vi "禹山浊度校准.vi"() -> ()   [LabVIEW 2016, in "斯坦道多参数.lvlib"]
uses:
  <vilib>/Utility/miscctls.llb/LVPointTypeDef.ctl
  <vilib>/Analysis/NI_AALBase.lvlib
  <vilib>/Analysis/NI_AALPro.lvlib
  <vilib>/Utility/config.llb/NI_LVConfig.lvlib
panel:
  out "滤波设定":dbl
  out "通讯状态":string
  out "第二点校准值":dbl
  out "第一点校准值":dbl
  out "最小值":sgl format="%.2g"
  out "最大值":sgl format="%.2g"
  in  "校准停止":bool
  in  "校准模式":u16(ring) items=["两点校准", "单点校准"]
  in  "标液2":dbl
  in  "标液1":dbl
  out "波形图表":sgl(graph) caption="历史曲线"
  out "温度测量值":dbl caption="温度" format="%#.2f"
  out "变异系数":dbl format="%.6g"
  out "standard deviation":dbl caption="标准差" format="%0.2f"
  out "mean":dbl caption="均值" format="%0.2f"
  out "提示":string
  in  "校准启动":bool
  out "测试值":dbl format="%#.2f"
  out "电极斜率":dbl format="%#.6f"
  out "电极零点":dbl format="%#.6f"
  # "浊度电极设定"
  # "℃"
  # "NTU"
  # "请选择校准模式:"
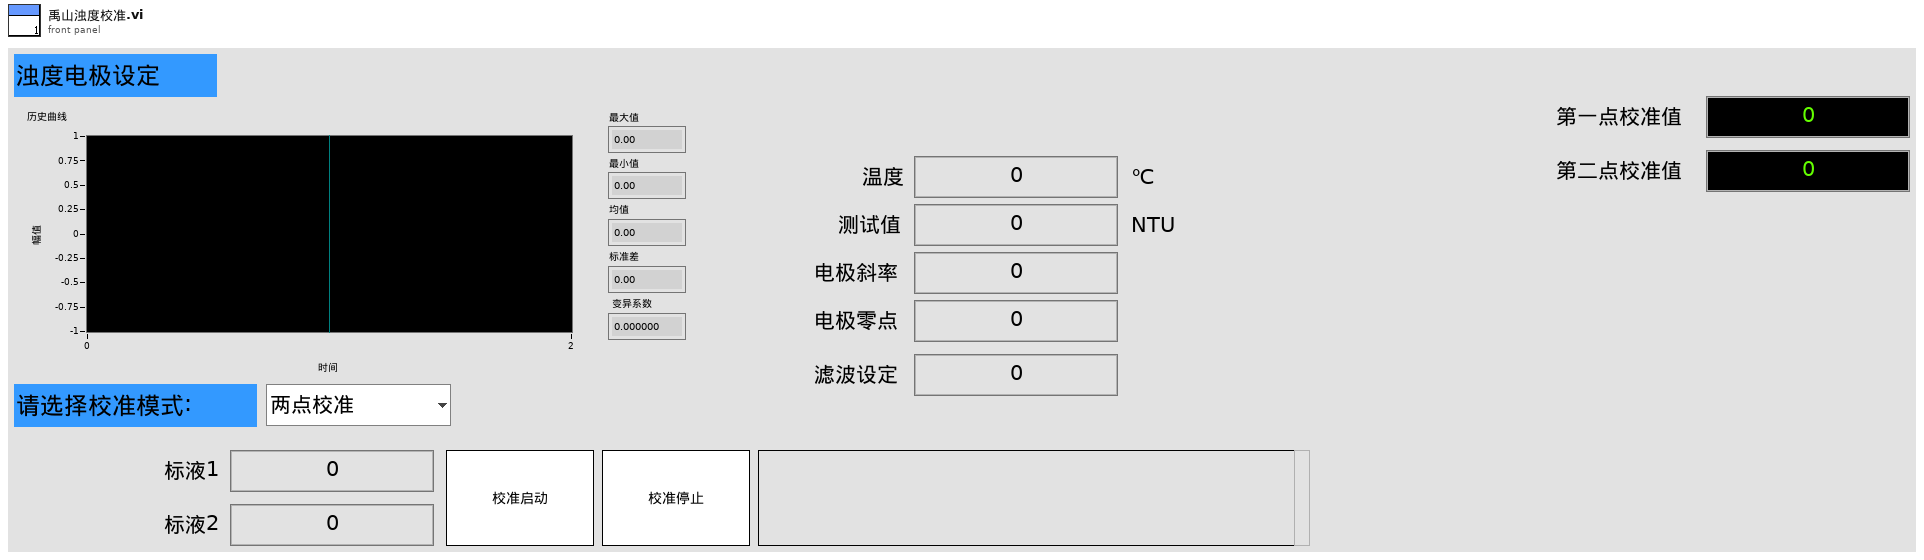
[diagram p1: front panel]
types:
  T1 = typedef "LVPointTypeDef.ctl" = cluster{"Horizontal":i16, "Vertical":i16}
  T2 = cluster{"pH":u32, "DO":u32, "Cond":u32, "Turb":u32, "叶绿素a":u32, "藻密度":u32, "ORP":u32}
  T3 = typedef "NI_LVConfig.lvlib/Config Data RefNum.ctl" = refnum<k1>
  T4 = enum8{"Enabled", "Disabled", "Disabled and Grayed Out"}
  T5 = cluster{"ph":bool, "DO":bool, "Cond":bool, "Turb":bool, "叶绿素a":bool, "藻密度":bool, "ORP":bool}
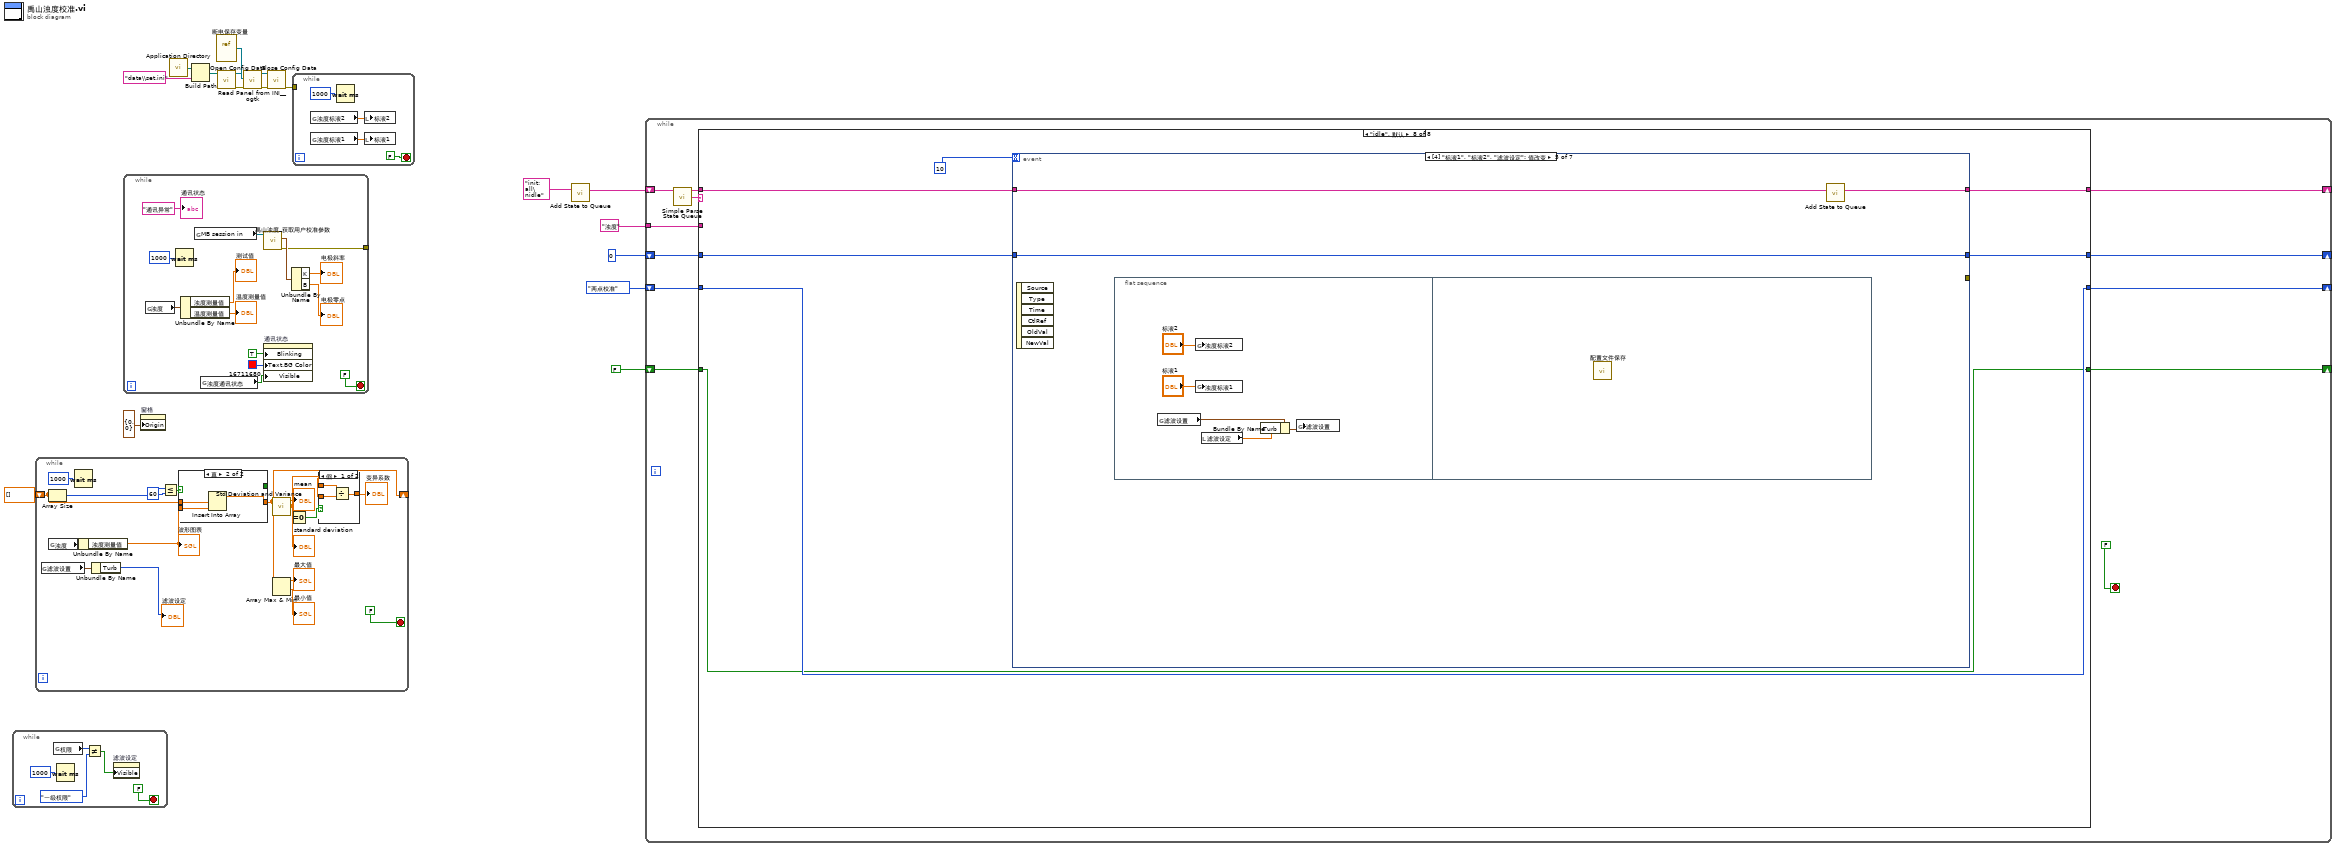
[diagram p0: block diagram]
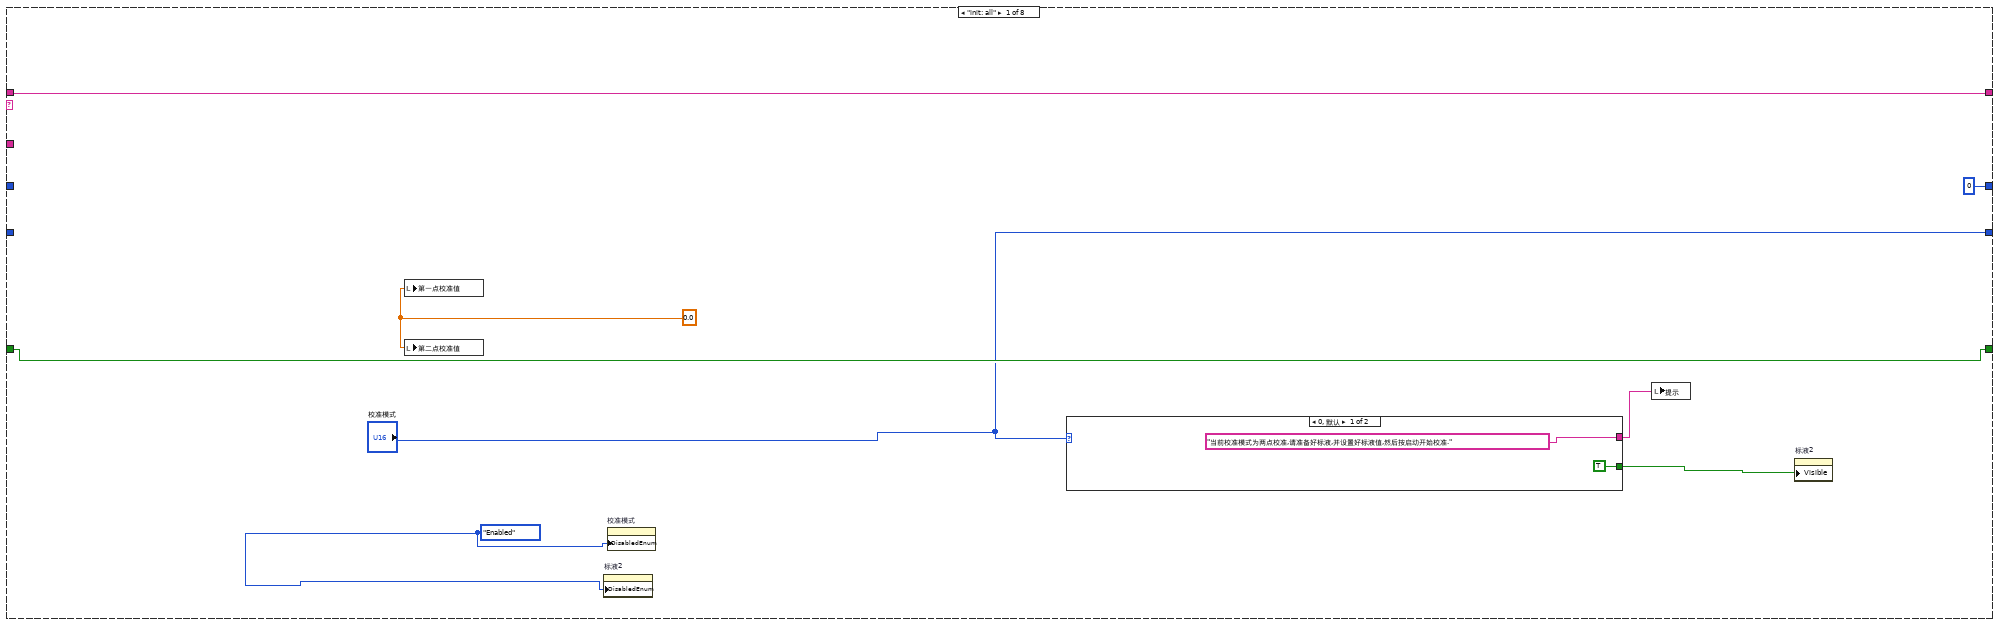
[diagram p2: hidden frame]
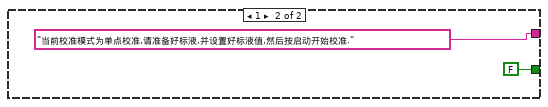
[diagram p3: hidden frame]
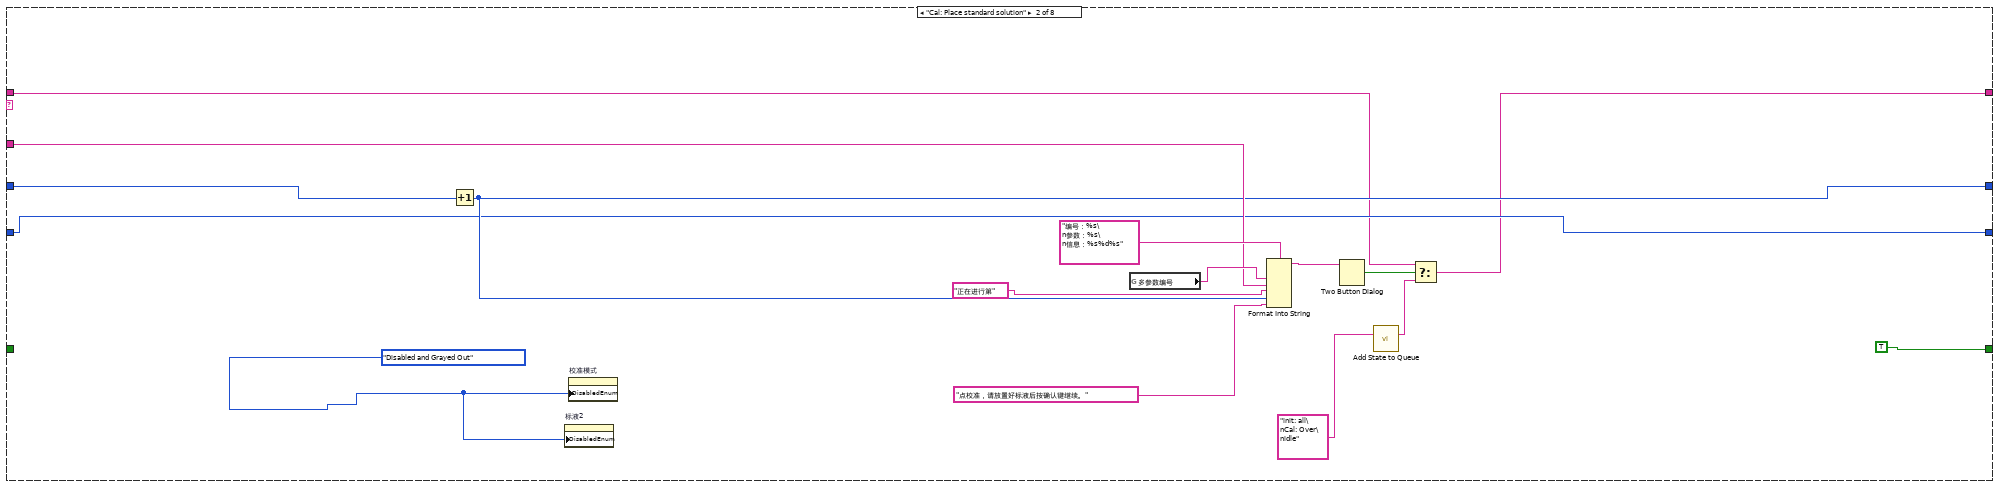
[diagram p4: hidden frame]
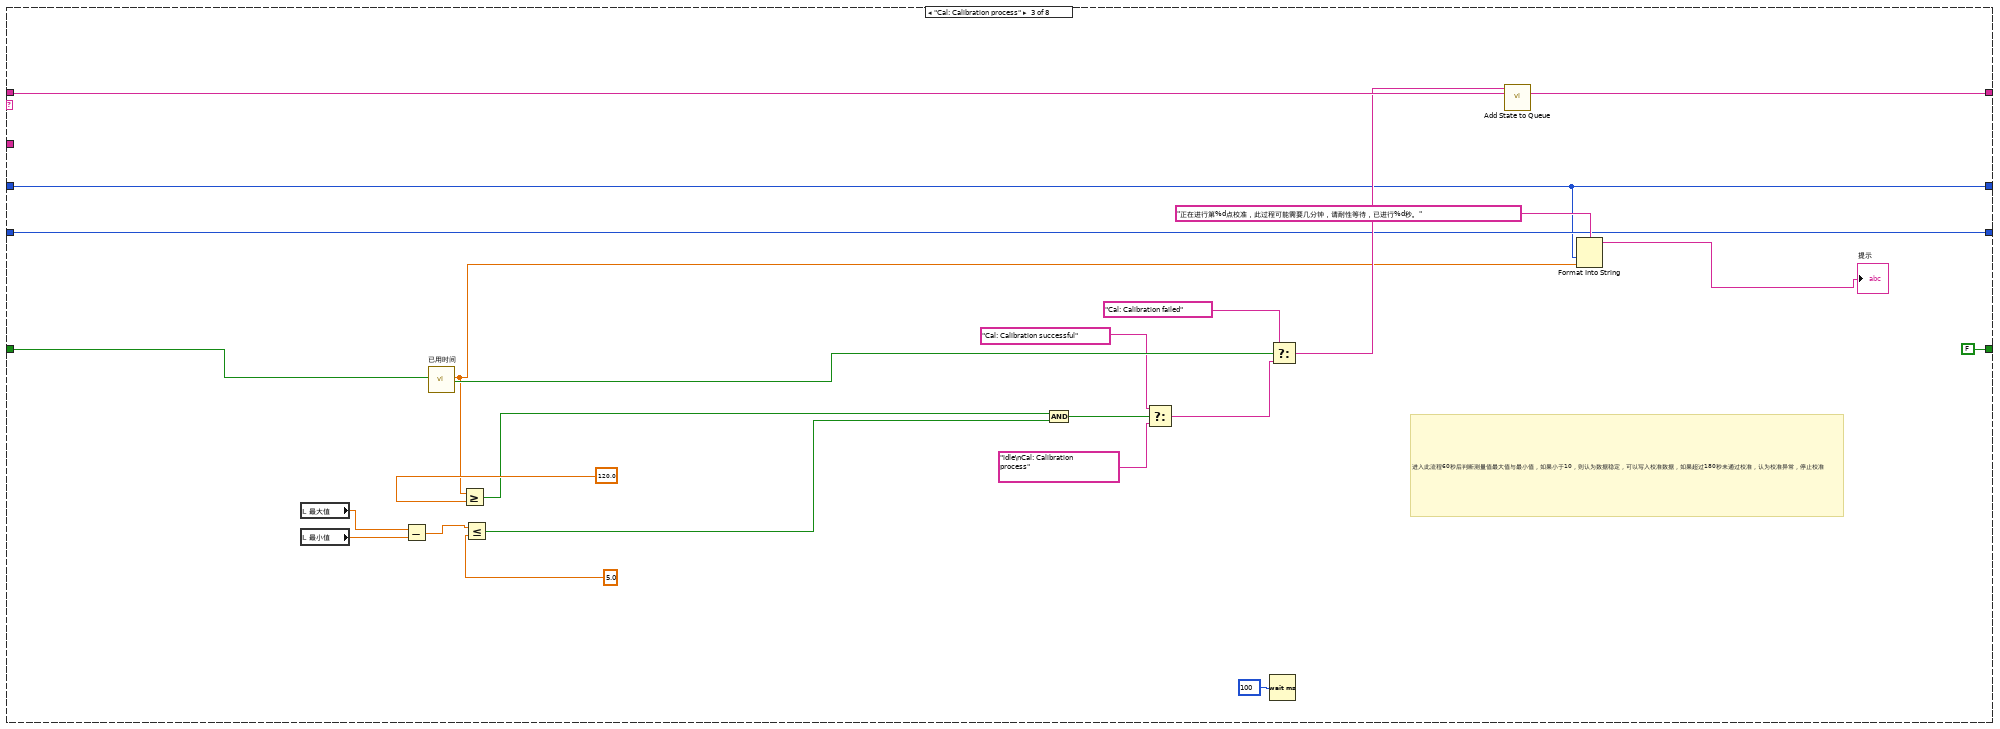
[diagram p5: hidden frame]
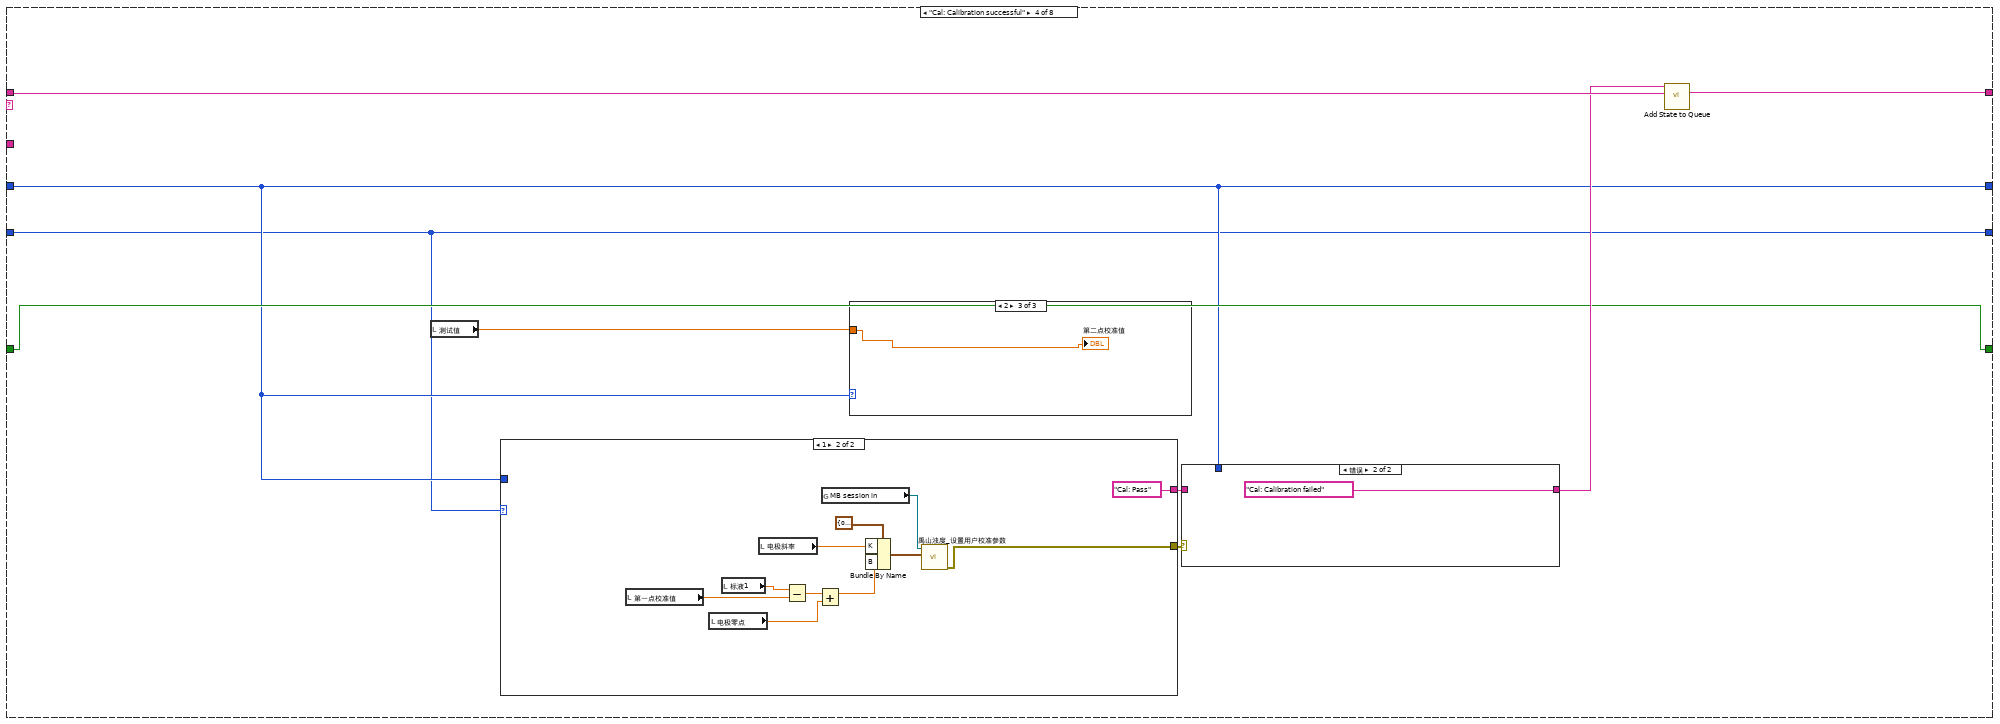
[diagram p6: hidden frame]
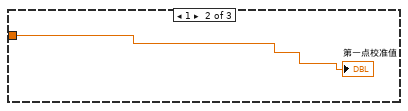
[diagram p8: hidden frame]
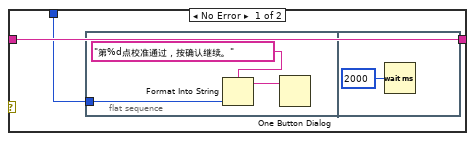
[diagram p9: hidden frame]
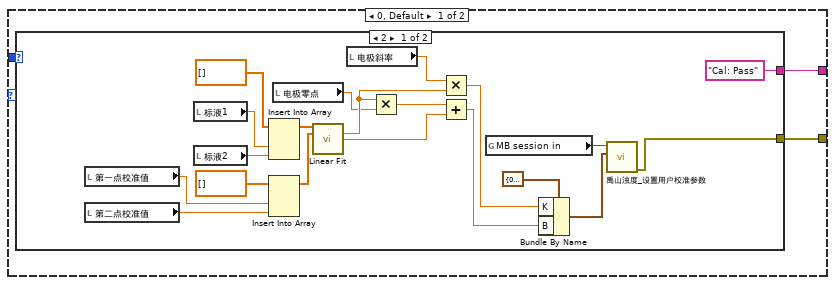
[diagram p10: hidden frame]
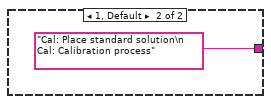
[diagram p11: hidden frame]
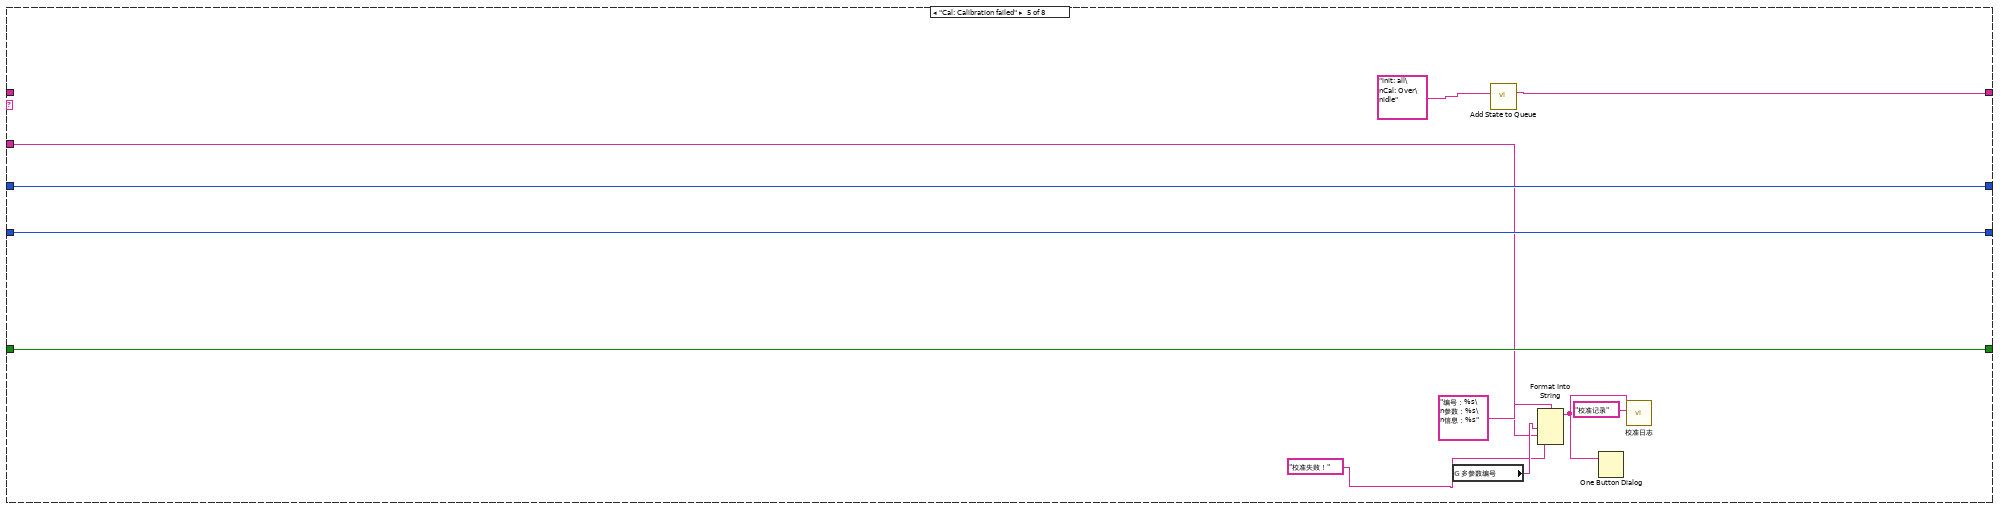
[diagram p12: hidden frame]
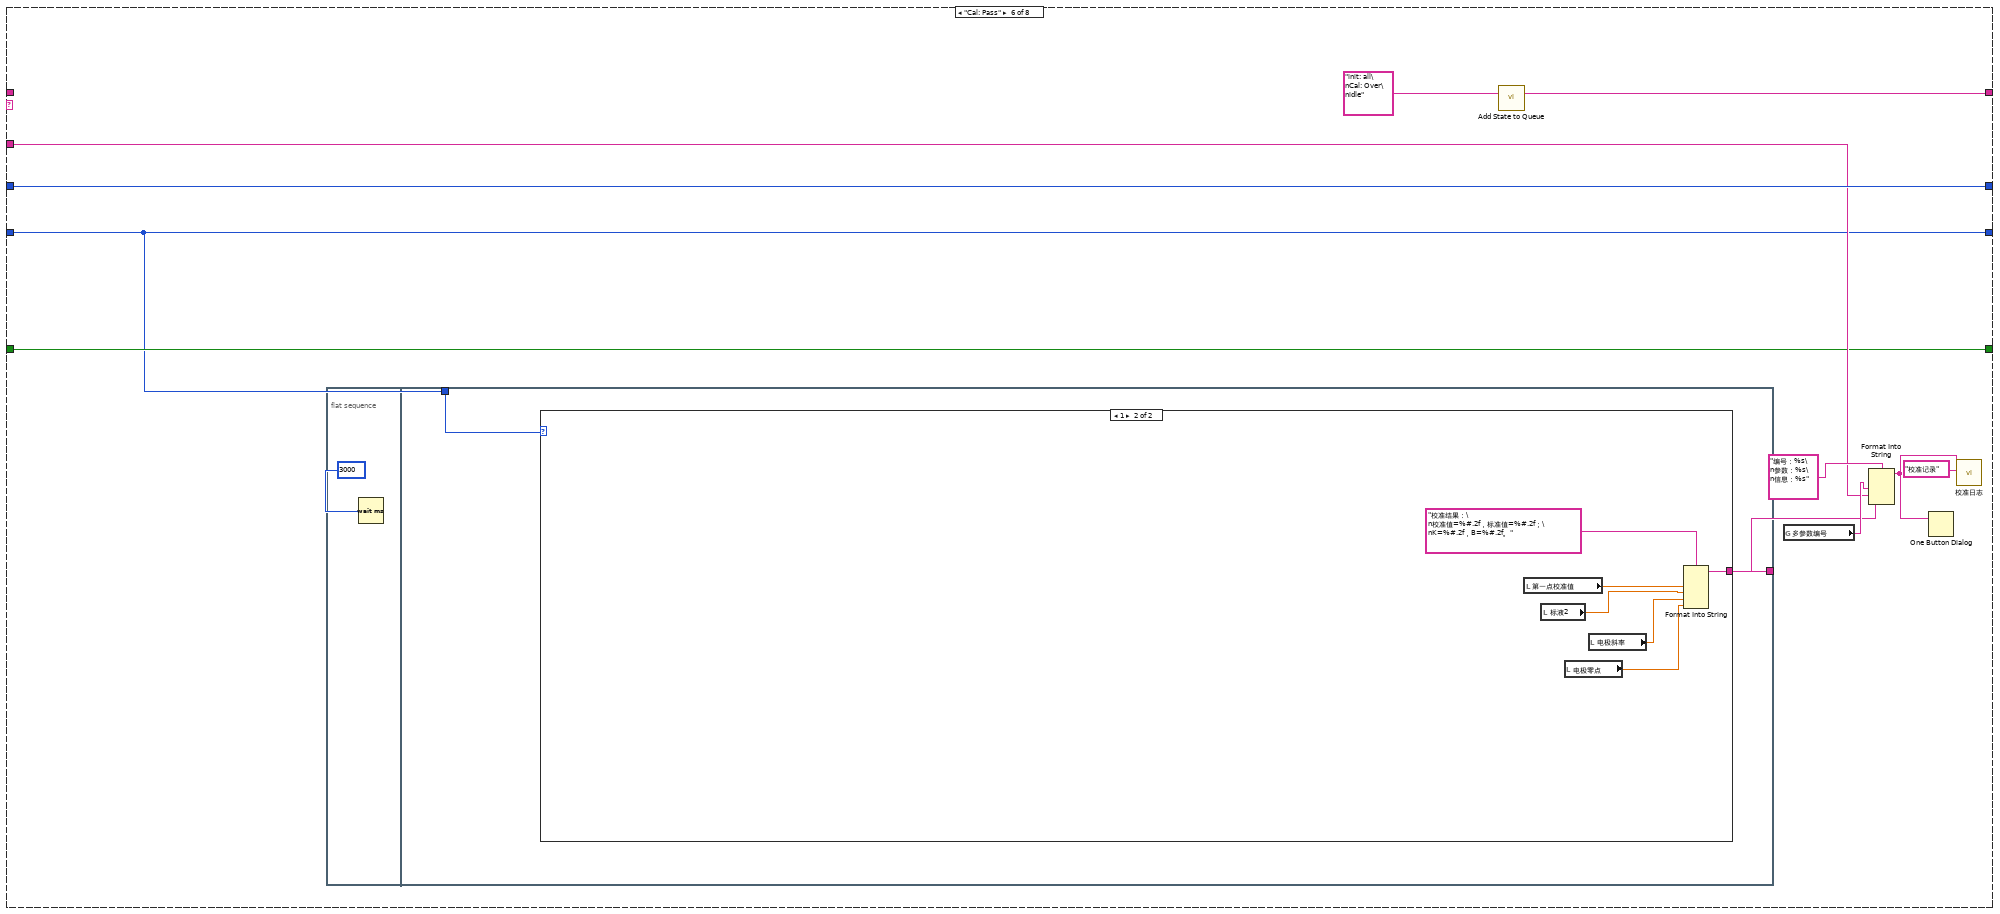
[diagram p13: hidden frame]
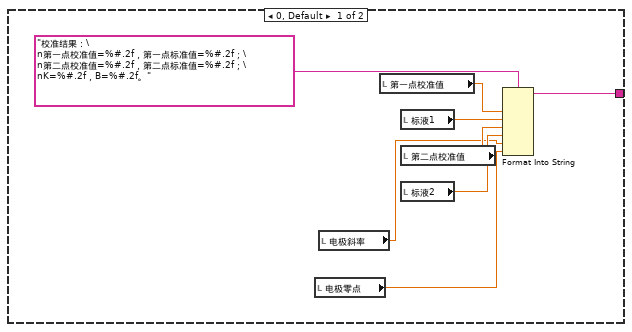
[diagram p14: hidden frame]
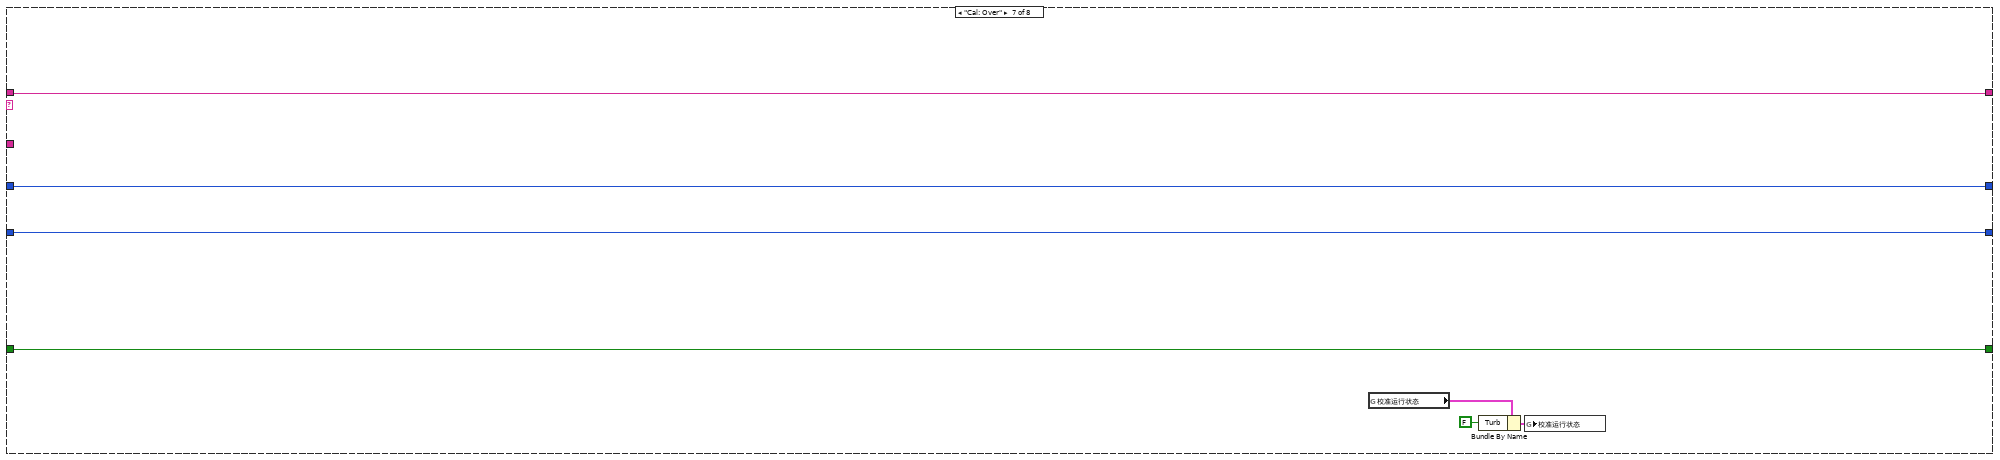
[diagram p15: hidden frame]
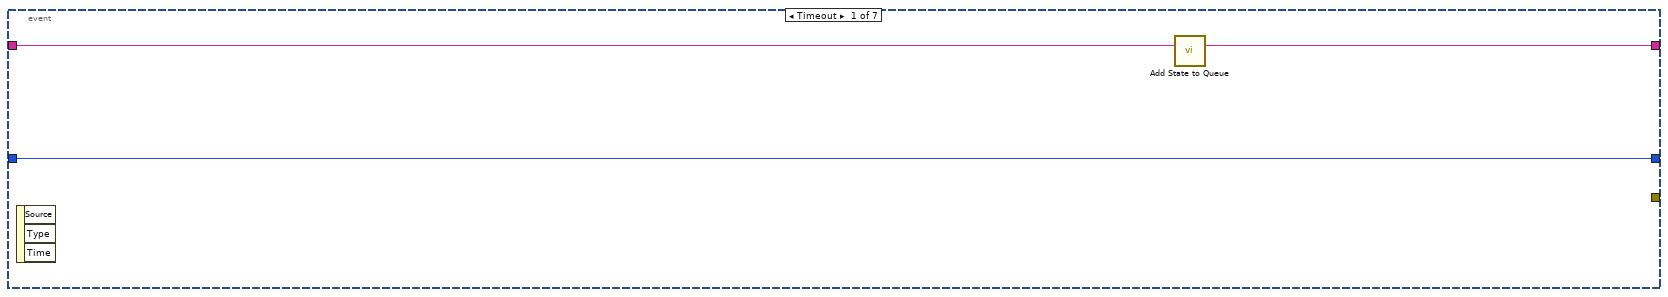
[diagram p16: hidden frame]
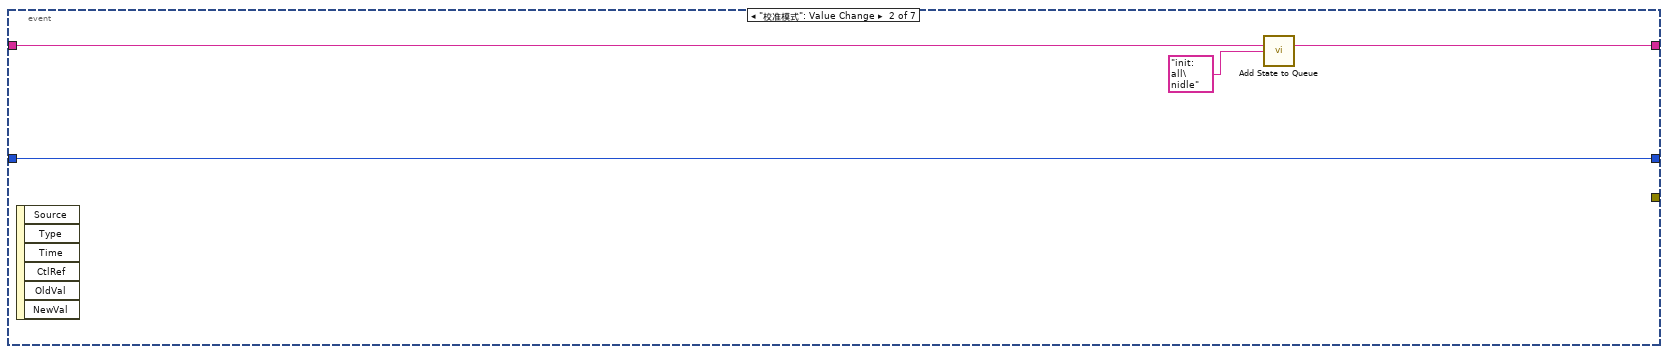
[diagram p17: hidden frame]
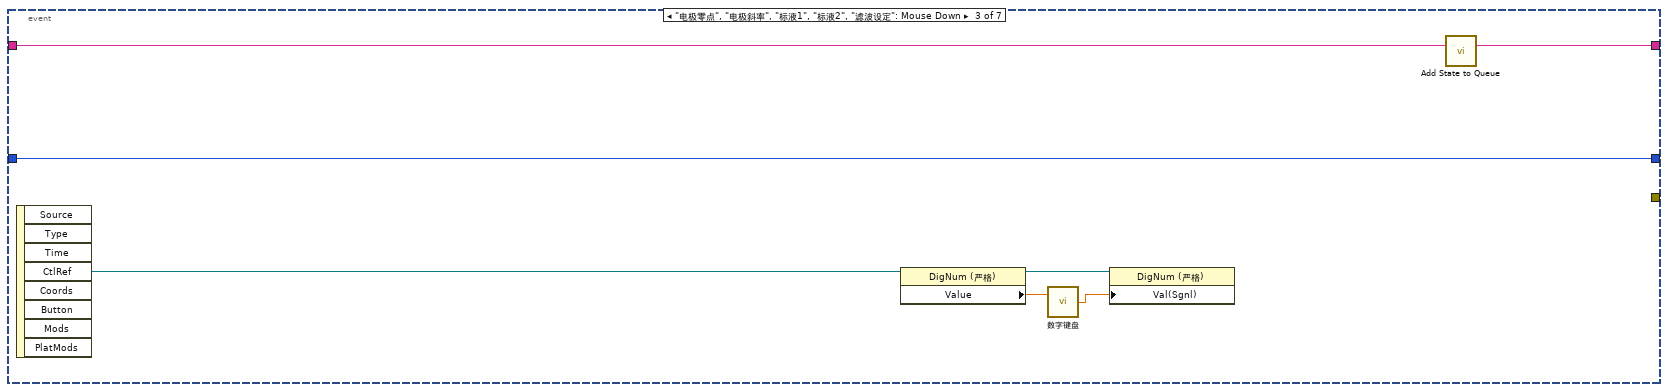
[diagram p18: hidden frame]
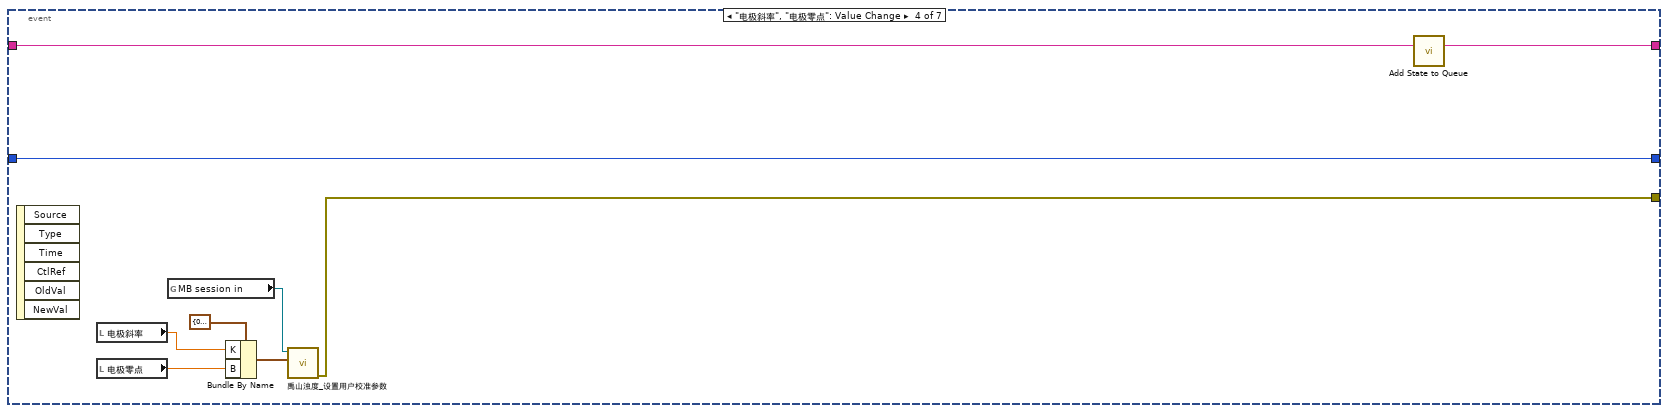
[diagram p19: hidden frame]
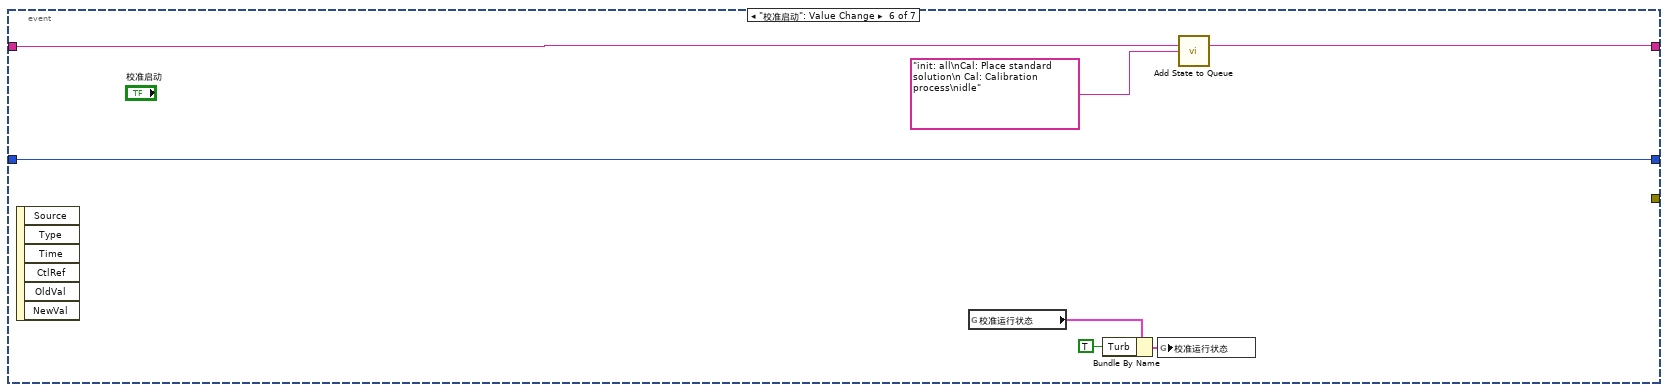
[diagram p20: hidden frame]
diagram:
  n1 = while {
    stop <- FALSE stop-if-true
    n2 = global read "多参数全局变量.vi" "权限"() -> (w21:enum16{"一级权限", "二级权限", "三级权限"})
    n3 = Wait (ms)(milliseconds to wait=u32 1000 ("等待时间（毫秒）")) -> ()  [unwired: 1 out]
    n4 = Not Equal?(x=w21, y=enum16{"一级权限", "二级权限", "三级权限"}."一级权限") -> (x != y?=w18:bool)
    n5 = property on="滤波设定" class="DigNum (严格)"("Visible"=w18) -> ()  [unwired: 2 in, 2 out]
  }
  n6 = while {
    shift-right: [w28] -> _
    shift-left: sgl[] [] -> [w35]
    stop <- FALSE stop-if-true
    n7 = global read "断电保存变量.vi" "滤波设置"() -> (w24:T2)
    n8 = Array Size(array=w35) -> (size(s)=w37:i32)
    n9 = global read "禹山过程全局变量.vi" "浊度"() -> (w29:cluster{"温度测量值":sgl, "浊度测量值":sgl})
    n10 = Wait (ms)(milliseconds to wait=u32 1000 ("等待时间（毫秒）")) -> ()  [unwired: 1 out]
    n11 = Unbundle By Name(w29) -> ("浊度测量值"=w25:sgl)
    "波形图表" <- w25
    n12 = Unbundle By Name(w24) -> ("Turb"=→"滤波设定":u32)
    n13 = Less Or Equal?(x=w37, y=60) -> (x <= y?=w36:bool)
    n14 = case shown="真" w36 {
      tunnel: w35 -> [w48 w51]
      tunnel: w25 -> [w46 w50]
      tunnel: [w44 w49] -> w28
      tunnel: [TRUE _] -> _
      frame False {
        n15 = Replace Array Subset(array=w48, new element=w46) -> (w47:sgl[])  [unwired: 1 in]
        n16 = Rotate 1D Array(1:w47, 2:-1 ("n")) -> (0:w44:sgl[])
      }
      frame True {
        n17 = Insert Into Array(array=w51, new element=w50) -> (w49:sgl[])  [unwired: 1 in]
      }
    }
    n18 = call <vilib>:"Std Deviation and Variance.vi"("X"=w28) -> ("mean"=w30:dbl, "standard deviation"=w31:dbl)  [unwired: 1 in, 1 out]
    "standard deviation" <- w31
    "mean" <- w30
    n19 = Array Max & Min(array=w28) -> (max value=→"最大值":sgl, min value=→"最小值":sgl)  [unwired: 2 out]
    n20 = Equal To 0?(x=w30) -> (x = 0?=w34:bool)
    n21 = case shown="假" w34 {
      tunnel: w31 -> [w42 _]
      tunnel: [w41 _] -> w33
      tunnel: w30 -> [w40 _]
      frame False {
        n22 = Divide(x=w42, y=w40) -> (x/y=w41:dbl)
      }
      frame True {
      }
    }
    "变异系数" <- w33
  }
  n23 = while {
    tunnel: [w60] -> _
    stop <- FALSE stop-if-true
    n24 = global read "禹山过程全局变量.vi" "浊度"() -> (w57:cluster{"温度测量值":sgl, "浊度测量值":sgl})
    n25 = Wait (ms)(milliseconds to wait=u32 1000 ("等待时间（毫秒）")) -> ()  [unwired: 1 out]
    n26 = Unbundle By Name(w57) -> ("浊度测量值"=→"测试值":sgl, "温度测量值"=→"温度测量值":sgl)
    n27 = global read "多参数全局变量.vi" "MB session in"() -> (w56:refnum<class "MB_Master.lvclass">)
    n28 = global read "多参数全局变量.vi" "浊度通讯状态"() -> (w52:bool)
    n29 = call "禹山浊度_获取用户校准参数.vi"("MB session in"=w56) -> ("error out"=w60:errorcluster, "输出值"=w63:cluster{"K":sgl, "B":sgl})  [unwired: 8 in, 1 out]
    n30 = property on="通讯状态" class="Str"("Blinking"=TRUE ("闪烁"), "Text.BG Color"=u32 16711680, "Visible"=w52) -> ()  [unwired: 2 in, 2 out]
    n31 = Unbundle By Name(w63) -> ("K"=→"电极斜率":sgl, "B"=→"电极零点":sgl)
    "通讯状态" <- "通讯异常" ("当前串口")
  }
  n32 = property on="窗格" class="Pane"("Origin"=T1 {"Horizontal"=0, "Vertical"=0} ("原点")) -> ()  [unwired: 2 in, 2 out]
  n33 = call <vilib>:"Application Directory.vi"() -> ("Application Directory"=w12:path)
  n34 = Build Path(base path=w12, name or relative path="data\\set.ini" ("名称或相对路径")) -> (appended path=w13:path)
  n35 = vi-ref "断电保存变量.vi"() -> (w15:refnum<vi>)
  n36 = call <vilib>:"Open Config Data.vi"("configuration file path"=w13) -> ("error out"=w9:errorcluster, "refnum"=w8:T3)  [unwired: 8 in, 1 out]
  n37 = call <userlib>:"Read Panel from INI__ogtk.vi"("error in (no error)"=w9, "VI ref"=w15, "refnum"=w8) -> ("error out"=w11:errorcluster, "refnum out"=w10:T3)  [unwired: 7 in]
  n38 = call <vilib>:"Close Config Data.vi"("error in (no error)"=w11, "refnum"=w10) -> ("error out"=w7:errorcluster)  [unwired: 8 in, 1 out]
  n39 = while {
    tunnel: w7 -> [_]
    stop <- FALSE stop-if-true
    n40 = global read "断电保存变量.vi" "浊度标液2"() -> (w66:dbl)
    n41 = global read "断电保存变量.vi" "浊度标液1"() -> (w67:dbl)
    n42 = Wait (ms)(milliseconds to wait=u32 1000 ("等待时间（毫秒）")) -> ()  [unwired: 1 out]
    n43 = local write "标液2"(w66) -> ()
    n44 = local write "标液1"(w67) -> ()
  }
  n45 = call "Add State to Queue.vi"("State(s) In (\"\")"="init: all\nidle" ("State(s) In (\"\")")) -> ("States Out"=w5:string)  [unwired: 14 in]
  n46 = while {
    shift-right: [w77] -> _
    shift-left: w5 -> [w81]
    shift-right: [w74] -> _
    shift-left: 0 -> [w76]
    tunnel: "浊度" ("State(s) In (\"\")") -> [w75]
    shift-right: [w72] -> _
    shift-left: enum16{"两点校准", "单点校准"}."两点校准" ("校准模式") -> [w73]
    shift-right: [w70] -> _
    shift-left: FALSE -> [w71]
    stop <- FALSE stop-if-true
    n47 = call "Simple Parse State Queue.vi"("State Queue"=w81) -> ("Remain States"=w78:string, "Next State"=w79:string)  [unwired: 13 in]
    n48 = case shown="\"idle\", 默认" w79 {
      tunnel: w78 -> [w89 w97 w128 w140 _ _ w232 w239]
      tunnel: [w89 w96 w127 w139 w194 w199 w232 w238] -> w77
      tunnel: w76 -> [_ w105 w112 w135 w197 w208 w231 w236]
      tunnel: w75 -> [_ w106 _ _ w188 w204 _ _]
      tunnel: [0 w103 w112 w135 w197 w208 w231 w237] -> w74
      tunnel: w73 -> [_ w102 w113 w134 w196 w200 w230 w235]
      tunnel: ["校准模式" w102 w113 w134 w196 w200 w230 w235] -> w72
      tunnel: w71 -> [w86 _ w115 w136 w195 w203 w229 w233]
      tunnel: [w86 TRUE FALSE w136 w195 w203 w229 w233] -> w70
      frame "init: all" {
        w85 = T4."Enabled" ("禁用")
        w82 = 0.0 ("第一点校准值")
        n49 = local write "第一点校准值"(w82) -> ()
        n50 = local write "第二点校准值"(w82) -> ()
        n51 = property on="标液2" class="DigNum (严格)"("DisabledEnum"=w85) -> ()  [unwired: 2 in, 2 out]
        n52 = property on="校准模式" class="Ring (严格)"("DisabledEnum"=w85) -> ()  [unwired: 2 in, 2 out]
        n53 = case shown="0, 默认" "校准模式" {
          tunnel: ["当前校准模式为两点校准,请准备好标液,并设置好标液值,然后按启动开始校准." ("提示") "当前校准模式为单点校准,请准备好标液,并设置好标液值,然后按启动开始校准." ("提示")] -> w88
          tunnel: [TRUE ("可见") FALSE ("可见")] -> w83
          frame 0, Default {
          }
          frame 1 {
          }
        }
        n54 = local write "提示"(w88) -> ()
        n55 = property on="标液2" class="DigNum (严格)"("Visible"=w83) -> ()  [unwired: 2 in, 2 out]
      }
      frame "Cal: Place standard solution" {
        w95 = T4."Disabled and Grayed Out" ("禁用")
        n56 = Increment(x=w105) -> (x+1=w103:i32)
        n57 = property on="标液2" class="DigNum (严格)"("DisabledEnum"=w95) -> ()  [unwired: 2 in, 2 out]
        n58 = property on="校准模式" class="Ring (严格)"("DisabledEnum"=w95) -> ()  [unwired: 2 in, 2 out]
        n59 = global read "多参数全局变量.vi" "多参数编号"() -> (w108:string)
        n60 = Format Into String(format string="编号：%s\n参数：%s\n信息：%s%d%s" ("格式字符串"), w108, w106, "正在进行第" ("消息"), w103, "点校准，请放置好标液后按确认键继续。" ("消息")) -> (resulting string=w100:string)  [unwired: 2 in, 1 out]
        n61 = Two Button Dialog(message=w100) -> (T button?=w99:bool)  [unwired: 2 in]
        n62 = call "Add State to Queue.vi"("State(s) In (\"\")"="init: all\nCal: Over\nidle" ("State(s) In (\"\")")) -> ("States Out"=w98:string)  [unwired: 14 in]
        n63 = Select(t=w97, s=w99, f=w98) -> (s? t:f=w96:string)
      }
      frame "Cal: Calibration process" {
        # "进入此流程60秒后判断测量值最大值与最小值，如果小于10，则认为数据稳定，可以写入校准数据，如果超过180秒未通过校准，认为校准异常，停止校准"
        n64 = local read "最大值"() -> (w132:sgl)
        n65 = local read "最小值"() -> (w131:sgl)
        n66 = Subtract(x=w132, y=w131) -> (x-y=w133:sgl)
        n67 = call "已用时间"("Reset"=w115) -> ("Elapsed Time (s)"=w111:dbl, "Time has Elapsed"=w129:bool)  [unwired: 11 in, 6 out]
        n68 = Greater Or Equal?(x=w111, y=120.0) -> (x >= y?=w124:bool)
        n69 = Less Or Equal?(x=w133, y=5.0) -> (x <= y?=w120:bool)
        n70 = And(x=w124, y=w120) -> (x .and. y?=w121:bool)
        n71 = Select(t="Cal: Calibration successful" ("State(s) In (\"\")"), s=w121, f="idle\nCal: Calibration process" ("State(s) In (\"\")")) -> (s? t:f=w119:string)
        n72 = Wait (ms)(milliseconds to wait=u32 100 ("等待时间（毫秒）")) -> ()  [unwired: 1 out]
        n73 = Select(t="Cal: Calibration failed" ("State(s) In (\"\")"), s=w129, f=w119) -> (s? t:f=w118:string)
        n74 = call "Add State to Queue.vi"("State(s) In Front (\"\")"=w118, "State(s) In (\"\")"=w128) -> ("States Out"=w127:string)  [unwired: 13 in]
        n75 = Format Into String(format string="正在进行第%d点校准，此过程可能需要几分钟，请耐性等待，已进行%d秒。" ("格式字符串"), w112, w111) -> (resulting string=→"提示":string)  [unwired: 2 in, 1 out]
      }
      frame "Cal: Calibration successful" {
        n76 = local read "测试值"() -> (w137:dbl)
        n77 = case shown="1" w134 {
          tunnel: [w154 w176] -> w142
          tunnel: [w153 "Cal: Pass" ("State(s) In (\"\")")] -> w141
          tunnel: w135 -> [w152 _]
          frame 0, Default {
            n78 = case shown="2" w152 {
              tunnel: [w155 _] -> w154
              tunnel: ["Cal: Pass" ("State(s) In (\"\")") "Cal: Place standard solution\n Cal: Calibration process" ("State(s) In (\"\")")] -> w153
              frame 2 {
                n79 = local read "第一点校准值"() -> (w172:dbl)
                n80 = local read "第二点校准值"() -> (w171:dbl)
                n81 = local read "标液1"() -> (w169:dbl)
                n82 = local read "标液2"() -> (w168:dbl)
                n83 = Insert Into Array(array=dbl[] [] ("Weight"), new element #1=w169, new element #2=w168) -> (w167:dbl[])  [unwired: 1 in]
                n84 = Insert Into Array(array=dbl[] [] ("Weight"), new element #1=w172, new element #2=w171) -> (w166:dbl[])  [unwired: 1 in]
                n85 = local read "电极零点"() -> (w159:dbl)
                n86 = call <vilib>:"Linear Fit.vi"("Y"=w167, "X"=w166) -> ("slope"=w160:dbl, "intercept"=w157:dbl)  [unwired: 9 in, 3 out]
                n87 = local read "电极斜率"() -> (w162:dbl)
                n88 = Multiply(x=w160, y=w159) -> (x*y=w158:dbl)
                n89 = Multiply(x=w162, y=w160) -> (x*y=w161:dbl)
                n90 = Add(x=w158, y=w157) -> (x+y=w156:dbl)
                n91 = global read "多参数全局变量.vi" "MB session in"() -> (w165:refnum<class "MB_Master.lvclass">)
                n92 = Bundle By Name(cluster=cluster{"K":sgl, "B":sgl} {"K"=0.0, "B"=0.0} ("用户校准参数"), "K"=w161, "B"=w156) -> (w164:cluster{"K":sgl, "B":sgl})
                n93 = call "禹山浊度_设置用户校准参数.vi"("用户校准参数"=w164, "MB session in"=w165) -> ("error out"=w155:errorcluster)  [unwired: 8 in, 1 out]
              }
              frame 1, Default {
              }
            }
          }
          frame 1 {
            n94 = local read "第一点校准值"() -> (w181:dbl)
            n95 = local read "电极零点"() -> (w185:dbl)
            n96 = local read "标液1"() -> (w182:dbl)
            n97 = local read "电极斜率"() -> (w180:dbl)
            n98 = Subtract(x=w182, y=w181) -> (x-y=w183:dbl)
            n99 = Add(x=w183, y=w185) -> (x+y=w184:dbl)
            n100 = global read "多参数全局变量.vi" "MB session in"() -> (w177:refnum<class "MB_Master.lvclass">)
            n101 = Bundle By Name(cluster=cluster{"K":sgl, "B":sgl} {"K"=0.0, "B"=0.0} ("用户校准参数"), "K"=w180, "B"=w184) -> (w178:cluster{"K":sgl, "B":sgl})
            n102 = call "禹山浊度_设置用户校准参数.vi"("用户校准参数"=w178, "MB session in"=w177) -> ("error out"=w176:errorcluster)  [unwired: 8 in, 1 out]
          }
        }
        n103 = case shown="2" w135 {
          tunnel: w137 -> [_ w143 w144]
          frame 0, Default {
          }
          frame 1 {
            "第一点校准值" <- w143
          }
          frame 2 {
            "第二点校准值" <- w144
          }
        }
        n104 = case shown="错误" w142 {
          tunnel: w141 -> [w146 _]
          tunnel: [w146 "Cal: Calibration failed" ("State(s) In (\"\")")] -> w138
          tunnel: w135 -> [w145 _]
          frame No Error {
            n105 = flat-sequence {
              tunnel: w145 -> [w147]
              frame #0 {
                n106 = Format Into String(format string="第%d点校准通过，按确认继续。" ("格式字符串"), w147) -> (resulting string=w149:string)  [unwired: 2 in, 1 out]
                n107 = One Button Dialog(message=w149) -> ()  [unwired: 1 in, 1 out]
              }
              frame #1 {
                n108 = Wait (ms)(milliseconds to wait=u32 2000 ("等待时间（毫秒）")) -> ()  [unwired: 1 out]
              }
            }
          }
          frame Error {
          }
        }
        n109 = call "Add State to Queue.vi"("State(s) In Front (\"\")"=w138, "State(s) In (\"\")"=w140) -> ("States Out"=w139:string)  [unwired: 13 in]
      }
      frame "Cal: Calibration failed" {
        n110 = global read "多参数全局变量.vi" "多参数编号"() -> (w191:string)
        n111 = call "Add State to Queue.vi"("State(s) In (\"\")"="init: all\nCal: Over\nidle" ("State(s) In (\"\")")) -> ("States Out"=w194:string)  [unwired: 14 in]
        n112 = Format Into String(format string="编号：%s\n参数：%s\n信息：%s" ("格式字符串"), w191, w188, "校准失败！" ("消息")) -> (resulting string=w190:string)  [unwired: 2 in, 1 out]
        n113 = One Button Dialog(message=w190) -> ()  [unwired: 1 in, 1 out]
        n114 = call "校准日志.vi"("table"="校准记录", "日志信息"=w190) -> ()  [unwired: 9 in, 1 out]
      }
      frame "Cal: Pass" {
        n115 = flat-sequence {
          tunnel: [w211] -> w201
          tunnel: w200 -> [w210]
          frame #0 {
            n116 = Wait (ms)(milliseconds to wait=u32 3000 ("等待时间（毫秒）")) -> ()  [unwired: 1 out]
          }
          frame #1 {
            n117 = case shown="1" w210 {
              tunnel: [w219 w225] -> w211
              frame 0, Default {
                n118 = local read "电极零点"() -> (w212:dbl)
                n119 = local read "电极斜率"() -> (w213:dbl)
                n120 = local read "第一点校准值"() -> (w217:dbl)
                n121 = local read "标液1"() -> (w218:dbl)
                n122 = local read "第二点校准值"() -> (w215:dbl)
                n123 = local read "标液2"() -> (w214:dbl)
                n124 = Format Into String(format string="校准结果：\n第一点校准值=%#.2f，第一点标准值=%#.2f；\n第二点校准值=%#.2f，第二点标准值=%#.2f；\nK=%#.2f，B=%#.2f。" ("提示"), w217, w218, w215, w214, w213, w212) -> (resulting string=w219:string)  [unwired: 2 in, 1 out]
              }
              frame 1 {
                n125 = local read "第一点校准值"() -> (w224:dbl)
                n126 = local read "标液2"() -> (w222:dbl)
                n127 = local read "电极零点"() -> (w220:dbl)
                n128 = local read "电极斜率"() -> (w221:dbl)
                n129 = Format Into String(format string="校准结果：\n校准值=%#.2f，标准值=%#.2f；\nK=%#.2f，B=%#.2f。" ("提示"), w224, w222, w221, w220) -> (resulting string=w225:string)  [unwired: 2 in, 1 out]
              }
            }
          }
        }
        n130 = call "Add State to Queue.vi"("State(s) In (\"\")"="init: all\nCal: Over\nidle" ("State(s) In (\"\")")) -> ("States Out"=w199:string)  [unwired: 14 in]
        n131 = global read "多参数全局变量.vi" "多参数编号"() -> (w205:string)
        n132 = Format Into String(format string="编号：%s\n参数：%s\n信息：%s" ("格式字符串"), w205, w204, w201) -> (resulting string=w202:string)  [unwired: 2 in, 1 out]
        n133 = One Button Dialog(message=w202) -> ()  [unwired: 1 in, 1 out]
        n134 = call "校准日志.vi"("table"="校准记录", "日志信息"=w202) -> ()  [unwired: 9 in, 1 out]
      }
      frame "Cal: Over" {
        n135 = global read "多参数全局变量.vi" "校准运行状态"() -> (w227:T5)
        n136 = Bundle By Name(cluster=w227, "Turb"=FALSE) -> (w228:T5)
        n137 = global write "多参数全局变量.vi" "校准运行状态"(w228) -> ()
      }
      frame "idle", Default {
        n138 = event shown="[4] \"标液1\", \"标液2\", \"滤波设定\": 值改变" {
          selector: _ -> [_ _ _ _ _ _ _]
          dyn-events: _ -> [_ _ _ _ _ _ _]
          timeout: 10 -> [_ _ _ _ _ _ _]
          tunnel: [_ _ _ w255 _ _ _] -> _
          tunnel: w239 -> [w242 w246 w251 w254 w263 w277 _]
          tunnel: [w241 w245 w252 w261 w264 w276 w279] -> w238
          tunnel: [w240 w243 w253 w262 w265 w274 w280] -> w237
          tunnel: w236 -> [w240 w243 w253 w262 w265 w274 w280]
          event Timeout {
            n139 = event-data() -> ()  [unwired: 1 in, 3 out]
            n140 = call "Add State to Queue.vi"("State(s) In (\"\")"=w242) -> ("States Out"=w241:string)  [unwired: 14 in]
          }
          event "校准模式": Value Change {
            n141 = event-data() -> ()  [unwired: 1 in, 6 out]
            n142 = call "Add State to Queue.vi"("State(s) In (\"\")"=w246, "State(s) At Back (\"\")"="init: all\nidle" ("State(s) In (\"\")")) -> ("States Out"=w245:string)  [unwired: 13 in]
          }
          event "电极零点", "电极斜率", "标液1", "标液2", "滤波设定": Mouse Down {
            n143 = event-data() -> ("CtlRef"=w250:refnum<vi>)  [unwired: 1 in, 7 out]
            n144 = property class="DigNum (严格)"(reference=w250) -> (reference out=w247:refnum<vi>, "Value"=w248:dbl)  [unwired: 1 in, 1 out]
            n145 = call "数字键盘.vi"("OldNumber"=w248) -> ("NewNumber"=w249:dbl)  [unwired: 1 in]
            n146 = property class="DigNum (严格)"(reference=w247, "Val(Sgnl)"=w249) -> ()  [unwired: 1 in, 2 out]
            n147 = call "Add State to Queue.vi"("State(s) In (\"\")"=w251) -> ("States Out"=w252:string)  [unwired: 14 in]
          }
          event "电极斜率", "电极零点": Value Change {
            n148 = event-data() -> ()  [unwired: 1 in, 6 out]
            n149 = local read "电极斜率"() -> (w258:dbl)
            n150 = local read "电极零点"() -> (w259:dbl)
            n151 = global read "多参数全局变量.vi" "MB session in"() -> (w260:refnum<class "MB_Master.lvclass">)
            n152 = Bundle By Name(cluster=cluster{"K":sgl, "B":sgl} {"K"=0.0, "B"=0.0} ("用户校准参数"), "K"=w258, "B"=w259) -> (w257:cluster{"K":sgl, "B":sgl})
            n153 = call "禹山浊度_设置用户校准参数.vi"("用户校准参数"=w257, "MB session in"=w260) -> ("error out"=w255:errorcluster)  [unwired: 8 in, 1 out]
            n154 = call "Add State to Queue.vi"("State(s) In (\"\")"=w254) -> ("States Out"=w261:string)  [unwired: 14 in]
          }
          event "标液1", "标液2", "滤波设定": Value Change {
            n155 = event-data() -> ()  [unwired: 1 in, 6 out]
            n156 = flat-sequence {
              frame #0 {
                n157 = global read "断电保存变量.vi" "滤波设置"() -> (w268:T2)
                n158 = global write "断电保存变量.vi" "浊度标液2"("标液2") -> ()
                n159 = global write "断电保存变量.vi" "浊度标液1"("标液1") -> ()
                n160 = local read "滤波设定"() -> (w266:dbl)
                n161 = Bundle By Name(cluster=w268, "Turb"=w266) -> (w267:T2)
                n162 = global write "断电保存变量.vi" "滤波设置"(w267) -> ()
              }
              frame #1 {
                n163 = call "配置文件保存.vi"() -> ()  [unwired: 12 in]
              }
            }
            n164 = call "Add State to Queue.vi"("State(s) In (\"\")"=w263) -> ("States Out"=w264:string)  [unwired: 14 in]
          }
          event "校准启动": Value Change {
            n165 = event-data() -> ()  [unwired: 1 in, 6 out]
            n166 = global read "多参数全局变量.vi" "校准运行状态"() -> (w272:T5)
            n167 = Bundle By Name(cluster=w272, "Turb"=TRUE) -> (w273:T5)
            n168 = global write "多参数全局变量.vi" "校准运行状态"(w273) -> ()
            n169 = call "Add State to Queue.vi"("State(s) In (\"\")"=w277, "State(s) At Back (\"\")"="init: all\nCal: Place standard solution\n Cal: Calibration process\nidle" ("State(s) In (\"\")")) -> ("States Out"=w276:string)  [unwired: 13 in]
          }
          event "校准停止": Value Change {
            n170 = event-data() -> ()  [unwired: 1 in, 6 out]
            n171 = call "Add State to Queue.vi"("State(s) In (\"\")"="init: all\nCal: Over\nidle" ("State(s) In (\"\")")) -> ("States Out"=w279:string)  [unwired: 14 in]
          }
        }
      }
    }
  }
